vi "in_2d interp xi yi vectors.vi"(6 "yi":dbl[](array[numeric]), 7 "method":i32(ring) items=["nearest", "bilinear", "bicubic", "bicubic spline"], 8 "xi":dbl[](array[numeric]), 9 "Y":dbl[](array[numeric]), 10 "X":dbl[](array[numeric]), 11 "Z":dbl[][](array[numeric])) -> (3 "zi":dbl[][](array[numeric]))   [LabVIEW 2018, in "NI_Gmath.lvlib"]
uses:
  NI_Gmath.lvlib
  A x Vector.vi
  Real Dot Product.vi
  Array To Matrix - RA2.vi
  <vilib>/Analysis/NI_AALBase.lvlib
  <vilib>/Analysis/NI_AALPro.lvlib
  NI_Matrix.lvlib
panel:
  # "Interpolate 2D"
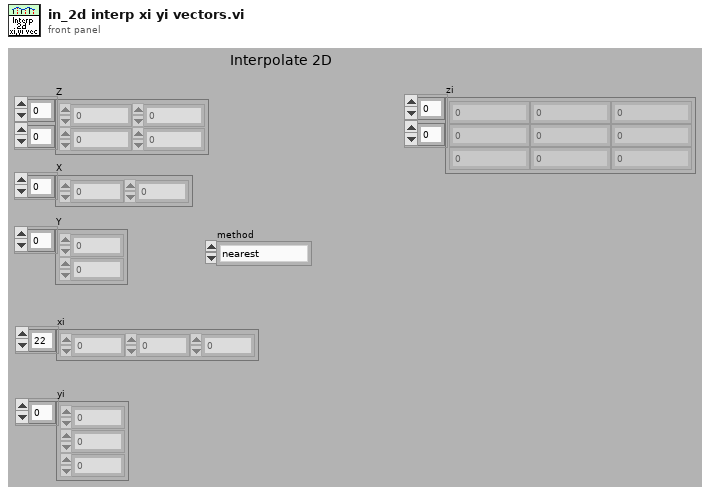
[diagram p1: front panel]
types:
  T1 = typedef "NI_Matrix.lvlib/RealMatrix.ctl" = dbl[][]
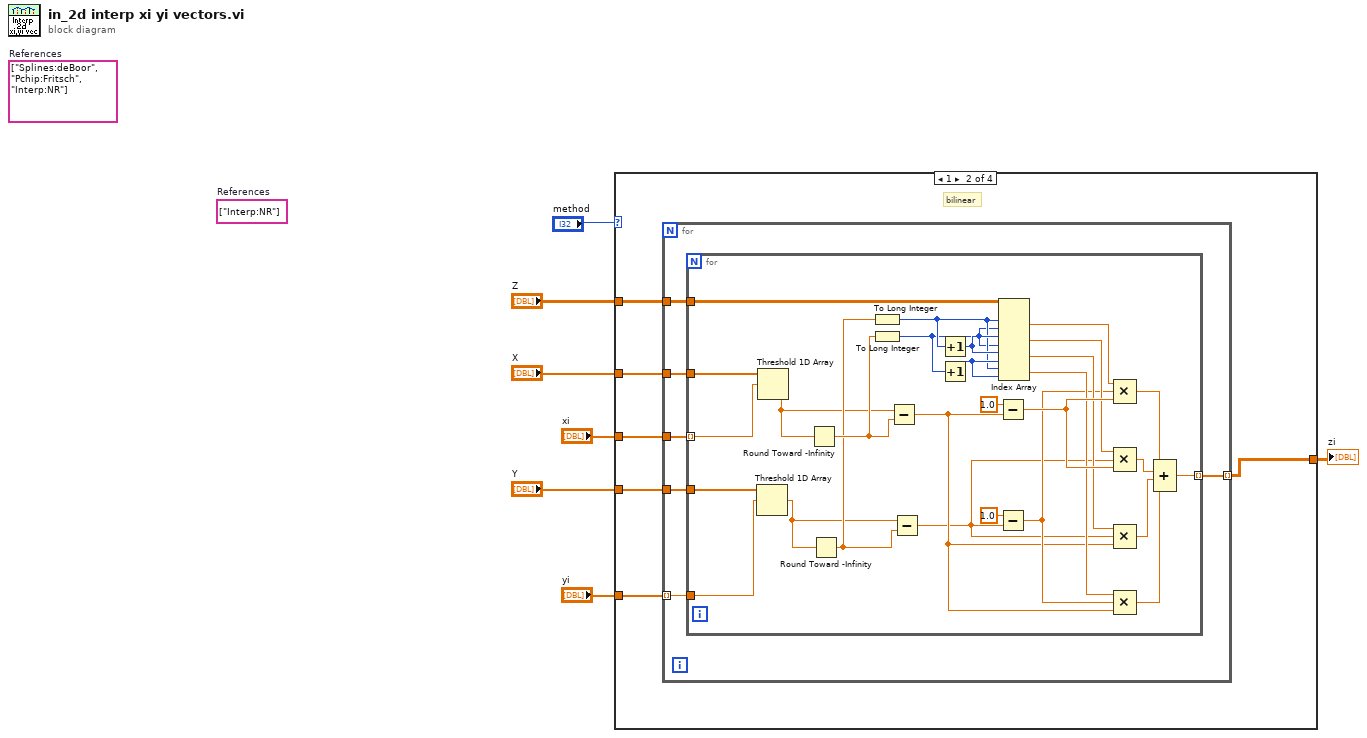
[diagram p0: block diagram]
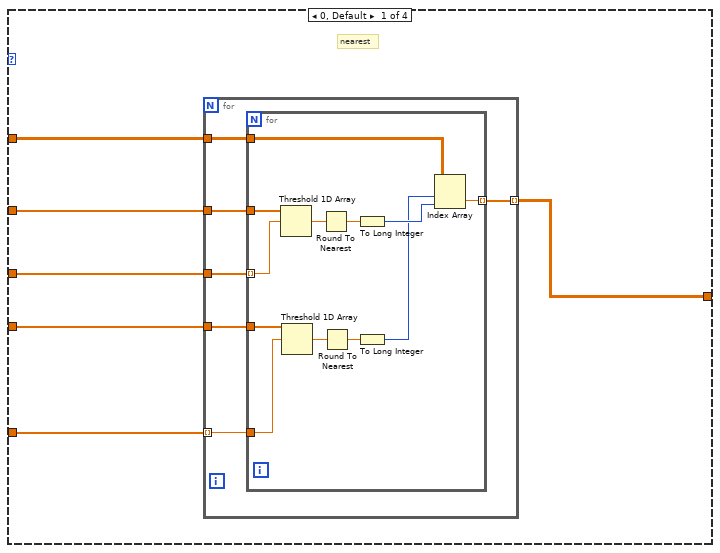
[diagram p2: hidden frame]
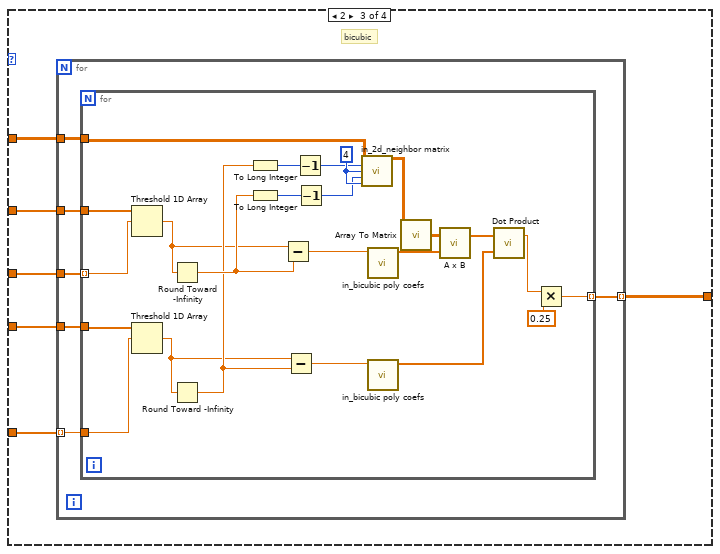
[diagram p3: hidden frame]
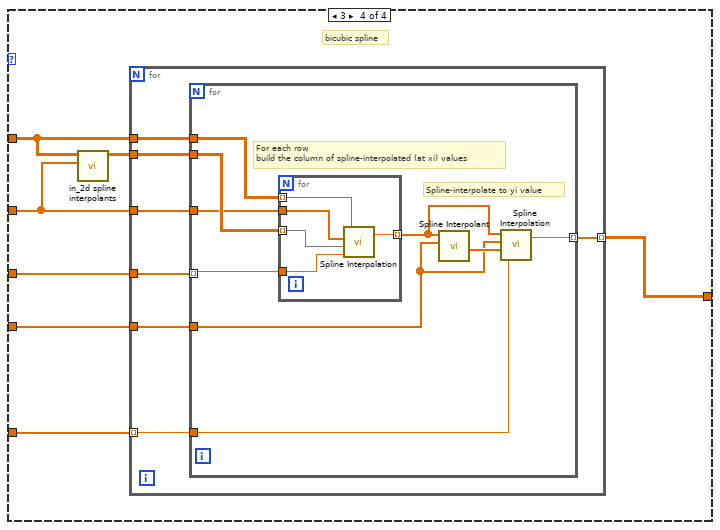
[diagram p4: hidden frame]
diagram:
  (unwired) string[] ["Interp:NR"]  # References
  (unwired) string[] ["Splines:deBoor", "Pchip:Fritsch", "Interp:NR"]  # References
  n1 = case shown="1" "method" {
    tunnel: "yi" -> [w13 w33 w73 w114]
    tunnel: "Y" -> [w12 w37 w77 w111]
    tunnel: "X" -> [w11 w36 w76 w109]
    tunnel: "Z" -> [w10 w35 w75 w110]
    tunnel: [w9 w32 w72 w112] -> w7
    tunnel: "xi" -> [w8 w34 w74 w108]
    frame 0, Default {
      # "nearest"
      n2 = for {
        tunnel: w12 -> [w15]
        tunnel: w13 -> [w14] mode=indexing
        tunnel: w11 -> [w19]
        tunnel: w10 -> [w18]
        tunnel: [w17] -> w9 mode=indexing
        tunnel: w8 -> [w16]
        n3 = for {
          tunnel: w19 -> [w30]
          tunnel: w18 -> [w29]
          tunnel: [w28] -> w17 mode=indexing
          tunnel: w16 -> [w24] mode=indexing
          tunnel: w15 -> [w26]
          tunnel: w14 -> [w25]
          n4 = Threshold 1D Array(2:w24, 3:w30) -> (0:w31:dbl)  [unwired: 1 in]
          n5 = Threshold 1D Array(2:w25, 3:w26) -> (0:w27:dbl)  [unwired: 1 in]
          n6 = Round To Nearest(number=w31) -> (nearest integer value=w23:dbl)
          n7 = Round To Nearest(number=w27) -> (nearest integer value=w21:dbl)
          n8 = To Long Integer(number=w23) -> (32bit integer=w22:i32)
          n9 = To Long Integer(number=w21) -> (32bit integer=w20:i32)
          n10 = Index Array(array=w29, index (row)=w20, index (col)=w22) -> (element=w28:dbl)
        }
      }
    }
    frame 1 {
      # "bilinear"
      n11 = for {
        tunnel: w37 -> [w43]
        tunnel: w36 -> [w42]
        tunnel: w35 -> [w41]
        tunnel: w34 -> [w40]
        tunnel: w33 -> [w39] mode=indexing
        tunnel: [w38] -> w32 mode=indexing
        n12 = for {
          tunnel: w43 -> [w71]
          tunnel: w39 -> [w57]
          tunnel: w42 -> [w53]
          tunnel: w41 -> [w70]
          tunnel: w40 -> [w46] mode=indexing
          tunnel: [w58] -> w38 mode=indexing
          n13 = Threshold 1D Array(2:w57, 3:w71) -> (0:w45:dbl)  [unwired: 1 in]
          n14 = Threshold 1D Array(2:w46, 3:w53) -> (0:w44:dbl)  [unwired: 1 in]
          n15 = Round Toward -Infinity(1:w44) -> (0:w50:dbl)
          n16 = Round Toward -Infinity(1:w45) -> (0:w47:dbl)
          n17 = To Long Integer(number=w47) -> (32bit integer=w55:i32)
          n18 = To Long Integer(number=w50) -> (32bit integer=w54:i32)
          n19 = Subtract(x=w44, y=w50) -> (x-y=w49:dbl)
          n20 = Subtract(x=w45, y=w47) -> (x-y=w48:dbl)
          n21 = Increment(x=w55) -> (x+1=w69:i32)
          n22 = Increment(x=w54) -> (x+1=w68:i32)
          n23 = Subtract(x=1.0, y=w49) -> (x-y=w64:dbl)
          n24 = Subtract(x=1.0, y=w48) -> (x-y=w51:dbl)
          n25 = Index Array(array=w70, index (row) #1=w55, index (col) #1=w54, index (row) #2=w69, index (col) #2=w54, index (row) #3=w69, index (col) #3=w68, index (row) #4=w55, index (col) #4=w68) -> (element #1=w65:dbl, element #2=w52:dbl, element #3=w63:dbl, element #4=w62:dbl)
          n26 = Compound Arithmetic op=MULTIPLY(w65, w51, w64) -> (w61:dbl)
          n27 = Compound Arithmetic op=MULTIPLY(w52, w48, w64) -> (w60:dbl)
          n28 = Compound Arithmetic op=MULTIPLY(w63, w48, w49) -> (w56:dbl)
          n29 = Compound Arithmetic op=MULTIPLY(w62, w51, w49) -> (w59:dbl)
          n30 = Compound Arithmetic op=ADD(w61, w60, w56, w59) -> (w58:dbl)
        }
      }
    }
    frame 2 {
      # "bicubic"
      n31 = for {
        tunnel: w77 -> [w83]
        tunnel: w76 -> [w82]
        tunnel: w75 -> [w81]
        tunnel: w74 -> [w80]
        tunnel: w73 -> [w79] mode=indexing
        tunnel: [w78] -> w72 mode=indexing
        n32 = for {
          tunnel: w83 -> [w107]
          tunnel: w79 -> [w99]
          tunnel: w82 -> [w106]
          tunnel: w81 -> [w105]
          tunnel: w80 -> [w100] mode=indexing
          tunnel: [w102] -> w78 mode=indexing
          w104 = 4 ("row length")
          n33 = Threshold 1D Array(2:w100, 3:w106) -> (0:w85:dbl)  [unwired: 1 in]
          n34 = Threshold 1D Array(2:w99, 3:w107) -> (0:w84:dbl)  [unwired: 1 in]
          n35 = Round Toward -Infinity(1:w85) -> (0:w89:dbl)
          n36 = Round Toward -Infinity(1:w84) -> (0:w86:dbl)
          n37 = To Long Integer(number=w86) -> (32bit integer=w92:i32)
          n38 = To Long Integer(number=w89) -> (32bit integer=w93:i32)
          n39 = Subtract(x=w85, y=w89) -> (x-y=w88:dbl)
          n40 = Subtract(x=w84, y=w86) -> (x-y=w87:dbl)
          n41 = Decrement(x=w92) -> (x-1=w91:i32)
          n42 = Decrement(x=w93) -> (x-1=w90:i32)
          n43 = call "in_2d_neighbor matrix.vi"("array"=w105, "row index"=w91, "row length"=w104, "col index"=w90, "col length"=w104) -> ("subarray"=w98:dbl[][])  [unwired: 10 in]
          n44 = call "in_bicubic poly coefs.vi"("t"=w88) -> ("bicubic polynomial"=w95:dbl[])  [unwired: 10 in]
          n45 = call "in_bicubic poly coefs.vi"("t"=w87) -> ("bicubic polynomial"=w96:dbl[])  [unwired: 10 in]
          n46 = call-poly "Array To Matrix.vi"("Real 2D Array"=w98) -> ("Real Matrix"=w94:T1)
          n47 = call-poly "A x B.vi"("Vector"=w95, "A"=w94) -> ("A x Vector"=w97:dbl[])  [unwired: 1 out]
          n48 = call-poly "Dot Product.vi"("Y Vector"=w96, "X Vector"=w97) -> ("X * Y"=w103:dbl)  [unwired: 1 out]
          n49 = Multiply(x=w103, y=0.25) -> (x*y=w102:dbl)
        }
      }
    }
    frame 3 {
      # "bicubic spline"
      n50 = call "in_2d spline interpolants.vi"("X row"=w109, "Z matrix"=w110) -> ("2d spline interpolants"=w113:dbl[][])  [unwired: 9 in]
      n51 = for {
        tunnel: w111 -> [w121]
        tunnel: w110 -> [w116]
        tunnel: w114 -> [w120] mode=indexing
        tunnel: w113 -> [w118]
        tunnel: w108 -> [w119]
        tunnel: w109 -> [w117]
        tunnel: [w115] -> w112 mode=indexing
        n52 = for {
          tunnel: w121 -> [w123]
          tunnel: w120 -> [w122]
          tunnel: w119 -> [w124] mode=indexing
          tunnel: w118 -> [w130]
          tunnel: w117 -> [w125]
          tunnel: w116 -> [w129]
          tunnel: [w126] -> w115 mode=indexing
          # "Spline-interpolate to yi value"
          # "For each row\nbuild the column of spline-interpolated (at xi) values"
          n53 = for {
            tunnel: w130 -> [w135] mode=indexing
            tunnel: w129 -> [w134] mode=indexing
            tunnel: [w133] -> w127 mode=indexing
            tunnel: w125 -> [w132]
            tunnel: w124 -> [w131]
            n54 = call "Spline Interpolation.vi"("x value"=w131, "Interpolant"=w135, "X"=w132, "Y"=w134) -> ("interpolation value"=w133:dbl)  [unwired: 1 out]
          }
          n55 = call "Spline Interpolant.vi"("X"=w123, "Y"=w127) -> ("Interpolant"=w128:dbl[])  [unwired: 2 in, 1 out]
          n56 = call "Spline Interpolation.vi"("x value"=w122, "Interpolant"=w128, "X"=w123, "Y"=w127) -> ("interpolation value"=w126:dbl)  [unwired: 1 out]
        }
      }
    }
  }
  "zi" <- w7
